vi "Hours_To_Time.vi"(8 "End":timestamp, 9 "Start":timestamp) -> (3 "time interval":T1)   [LabVIEW 2016]
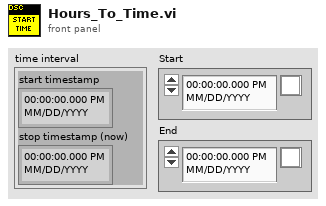
[diagram p1: front panel]
types:
  T1 = cluster{"start timestamp":timestamp, "stop timestamp (now)":timestamp}
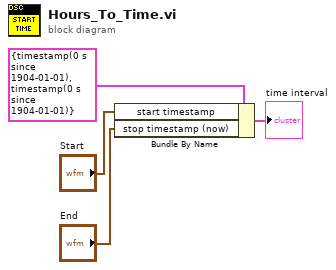
[diagram p0: block diagram]
diagram:
  n1 = Bundle By Name(cluster=T1 {"start timestamp"=timestamp(0 s since 1904-01-01), "stop timestamp (now)"=timestamp(0 s since 1904-01-01)} ("time interval"), "start timestamp"="Start", "stop timestamp (now)"="End") -> (→"time interval":T1)
